vi "SMTP_email_MultiAttach_Authenticated.vi"(0 "Recipients":string[](array[string]), 1 "timeout in ms (10000)":i32=10000, 2 "SMTPServer:Port":string, 5 "Subject":string, 7 "Message":string, 9 "Attachments":path[](array[path]), 11 "Error In":errorcluster, 12 "SMTP Credentials":T1, 13 "From Address":string) -> (4 "invalid recipients":string[](array[string]), 15 "Error Out":errorcluster)   [LabVIEW 2021]
uses:
  Utilities/Authentication/SMTPCredentials.ctl
  <vilib>/smtpClient/Set Message Text.vi
  <vilib>/smtpClient/LabVIEWSMTPClient.lvlib
panel:
  in  "Use Secure Connection (TLS\\SSL)":bool
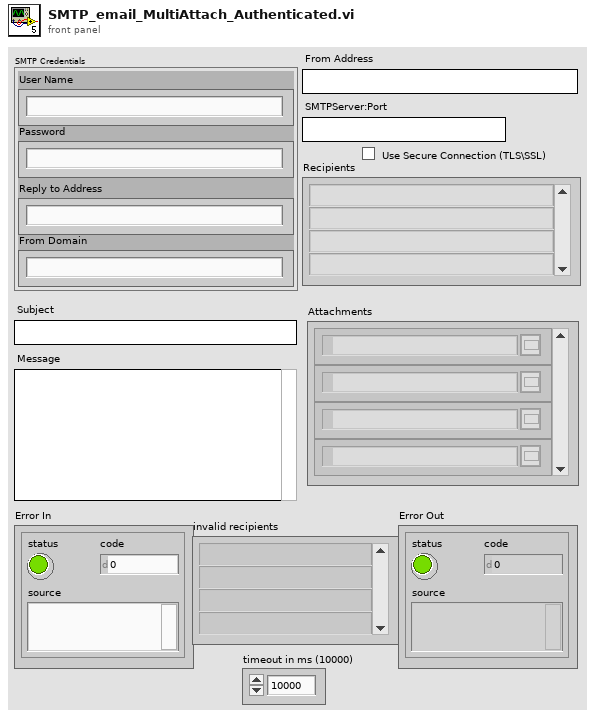
[diagram p1: front panel]
types:
  T1 = typedef "SMTPCredentials.ctl" = cluster{"User Name":string, "Password":string, "Reply to Address":string, "From Domain":string}
  T2 = typedef "LabVIEWSMTPClient.lvlib/SmtpClientHandle.ctl" = refnum<k1>
  T3 = cluster{"Name":string, "Reply to Address":string}
  T4 = cluster{"Name":string, "Reply to Address":string}[]
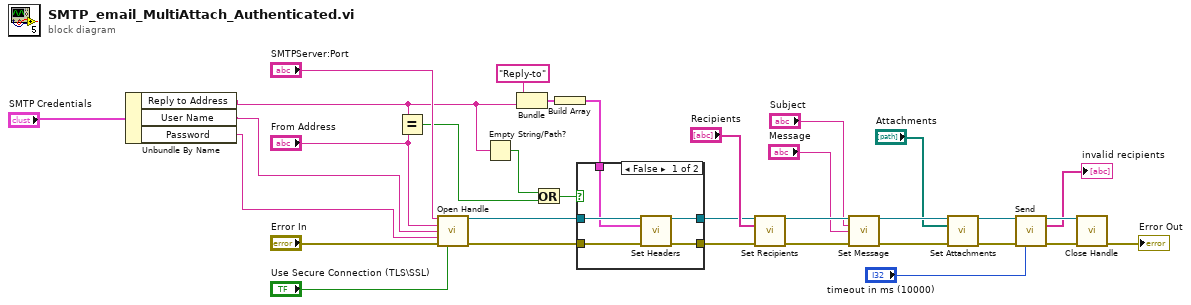
[diagram p0: block diagram]
diagram:
  n1 = Unbundle By Name("SMTP Credentials") -> ("Reply to Address"=w5:string, "User Name"=w4:string, "Password"=w3:string)
  n2 = Equal?(x=w5, y="From Address") -> (x = y?=w7:bool)
  n3 = call <vilib>:"Open Handle.vi"("server address"="SMTPServer:Port", "from"="From Address", "username"=w4, "password"=w3, "error in (no error)"="Error In", "use TLS (false)"="Use Secure Connection (TLS\\SSL)") -> ("handle out"=w15:T2, "error out"=w17:errorcluster)  [unwired: 8 in]
  n4 = Empty String/Path?(string/path=w5) -> (empty?=w10:bool)
  n5 = Bundle("Name"="Reply-to", "Reply to Address"=w5) -> (w12:T3)  [unwired: 1 in]
  n6 = Or(x=w10, y=w7) -> (x .or. y?=w9:bool)
  n7 = Build Array(w12) -> (w11:T4)
  n8 = case shown="False" w9 {
    tunnel: w17 -> [w38 w39]
    tunnel: [w37 w39] -> w16
    tunnel: w15 -> [w36 w40]
    tunnel: [w35 w40] -> w14
    tunnel: w11 -> [w34 _]
    frame False {
      n9 = call <vilib>:"Set Headers.vi"("handle in"=w36, "headers"=w34, "error in (no error)"=w38) -> ("handle out"=w35:T2, "error out"=w37:errorcluster)  [unwired: 11 in]
    }
    frame True {
    }
  }
  n10 = call <vilib>:"Set Recipients.vi"("handle in"=w14, "to"="Recipients", "error in (no error)"=w16) -> ("handle out"=w32:T2, "error out"=w31:errorcluster)  [unwired: 11 in]
  n11 = call-poly <vilib>:"Set Message.vi"("handle in"=w32, "subject"="Subject", "plain text message"="Message", "error in (no error)"=w31) -> ("handle out"=w26:T2, "error out"=w25:errorcluster)  [unwired: 10 in]
  n12 = call <vilib>:"Set Attachments.vi"("handle in"=w26, "attachments"="Attachments", "error in (no error)"=w25) -> ("handle out"=w24:T2, "error out"=w23:errorcluster)  [unwired: 11 in]
  n13 = call <vilib>:"Send.vi"("handle in"=w24, "error in (no error)"=w23, "timeout in ms (10000)"="timeout in ms (10000)") -> ("handle out"=w29:T2, "invalid recipients"=→"invalid recipients":string[], "error out"=w30:errorcluster)  [unwired: 10 in]
  n14 = call <vilib>:"Close Handle.vi"("handle in"=w29, "error in (no error)"=w30) -> ("error out"=→"Error Out":errorcluster)  [unwired: 12 in, 1 out]
